vi "Extract Channel Names and Addresses from Config.vi"(0 "Config":T1={"DAQ Settings"={"Trigger Type"=enum."Manual", "Trigger Samples"=0, "Pretrigger Samples"=0, "Trigger Interval"=0.0, "Time Units"=FALSE, "Auto Save"=FALSE, "Sample Rate"=7.0, "Select Analog"=FALSE, "Trigger Value"=0.0, "Trigger Stop Method"=enum."Use Samples Value to Stop Trigger", "Rate Sec/Min"=FALSE, "Save Mode"=enum."Single File", "File Size Limit"=0.0, "Log File Type"=enum."Basic", "Trigger Data Index"=0, "Log Rate"=7.0, "Rate Sec/Min (Log)"=FALSE, "Sample Rate (S/s)"=0.0, "Log Rate (S/s)"=0.0}, "Channels"=[], "Header"={"CA Number"="", "Test Name"="", "Serial Number"="", "Technician"=""}, "Graph Settings"={"Graph Labels"=[], [], [], [], [], [], [], [], [], [], [], [], [], "Graph Toggles"=[], "Axis Toggles"=[], "Graph Range"=enum."1"}, "Test Limits"=[], "All Type Info"=[], "Save Mode"=enum."Single File", "Data Base Path"=path ""} {"DAQ Settings"."Trigger Interval" min=0.0; "DAQ Settings"."Pretrigger Samples" min=0; "DAQ Settings"."Trigger Samples" min=0}) -> (4 "Channel Names":string[](array[string]), 6 "Channel Addresses":string[](array[string]))   [LabVIEW 2023]
uses:
  Type Defs and Controls/Sensor Config.ctl
  Type Defs and Controls/DAQ Settings.ctl
  Type Defs and Controls/Trigger Stop Method.ctl
  Type Defs and Controls/Log File Type.ctl
  Type Defs and Controls/Channel Config.ctl
  Type Defs and Controls/Header.ctl
  Type Defs and Controls/Graph Settings Type Def.ctl
  Type Defs and Controls/Test Limits.ctl
  Type Defs and Controls/All Part Info.ctl
  Type Defs and Controls/Part Info.ctl
panel:
  # "EGU"
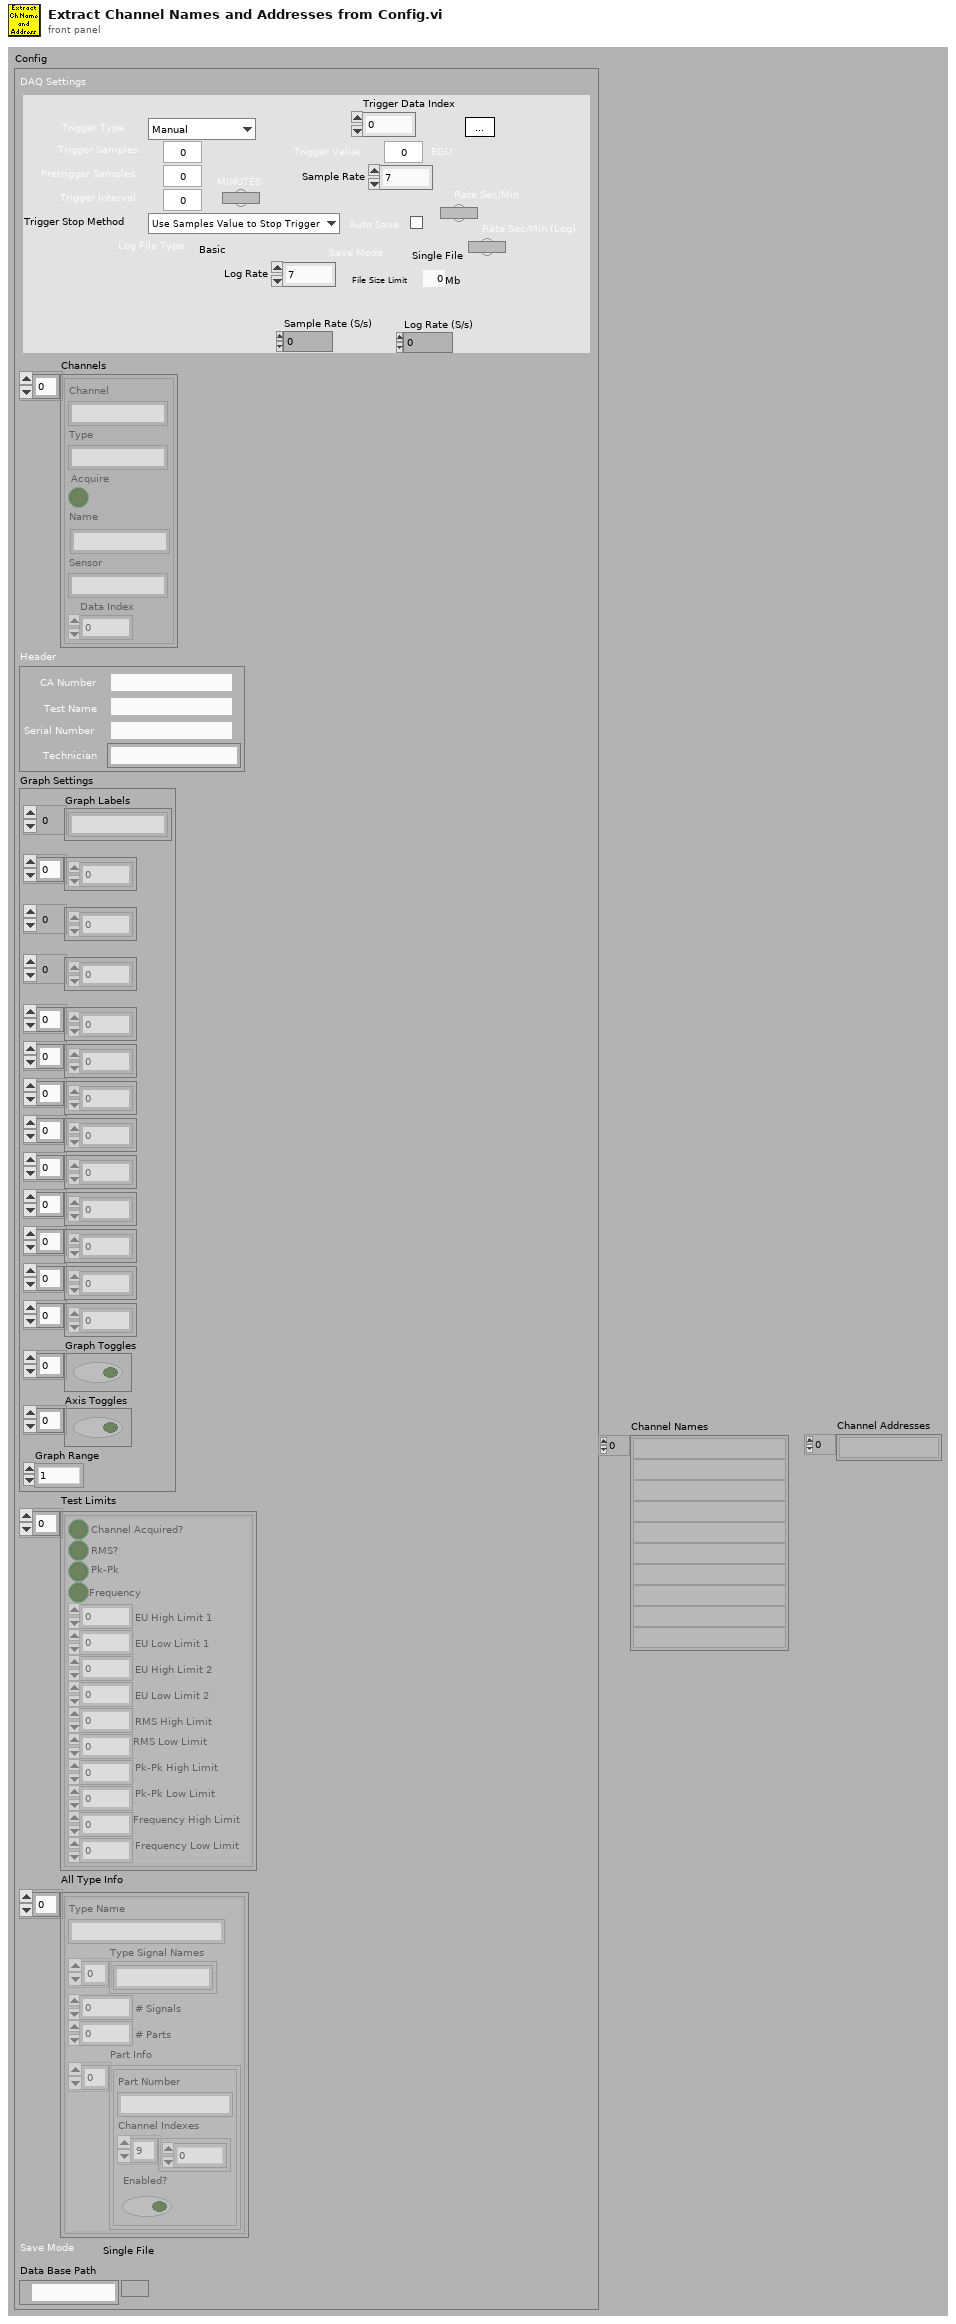
[diagram p1: front panel]
types:
  T1 = typedef "Sensor Config.ctl" = cluster{"DAQ Settings":T2, "Channels":T5[], "Header":T6, "Graph Settings":T7, "Test Limits":T8[], "All Type Info":T9, "Save Mode":enum16{"Single File", "Segmented Files", "New File at Midnight"}, "Data Base Path":path}
  T2 = typedef "DAQ Settings.ctl" = cluster{"Trigger Type":enum16{"Manual", "Timed", "Analog Rising", "Analog Falling"}, "Trigger Samples":i32, "Pretrigger Samples":i32, "Trigger Interval":dbl, "Time Units":bool, "Auto Save":bool, "Sample Rate":dbl, "Select Analog":bool, "Trigger Value":dbl, "Trigger Stop Method":T3, "Rate Sec/Min":bool, "Save Mode":enum16{"Single File", "Segmented Files", "New File at Midnight"}, "File Size Limit":dbl, "Log File Type":T4, "Trigger Data Index":u32, "Log Rate":dbl, "Rate Sec/Min (Log)":bool, "Sample Rate (S/s)":dbl, "Log Rate (S/s)":dbl}
  T3 = typedef "Trigger Stop Method.ctl" = enum16{"Use Samples Value to Stop Trigger", "Use Threshold to Stop Trigger"}
  T4 = typedef "Log File Type.ctl" = enum16{"Basic", "RTS"}
  T5 = typedef "Channel Config.ctl" = cluster{"Channel":string, "Type":string, "Acquire":bool, "Name":string, "Sensor":string, "Data Index":u32}
  T6 = typedef "Header.ctl" = cluster{"CA Number":string, "Test Name":string, "Serial Number":string, "Technician":string}
  T7 = typedef "Graph Settings Type Def.ctl" = cluster{"Graph Labels":string[], u8[], i16[], u32[], u8[], u8[], u8[], u32[], u8[], u8[], u8[], dbl[], dbl[], "Graph Toggles":bool[], "Axis Toggles":bool[], "Graph Range":enum16{"1", "2", "3", "4", "5", "10", "15", "30", "60"}}
  T8 = typedef "Test Limits.ctl" = cluster{"Channel Acquired?":bool, "RMS?":bool, "Pk-Pk":bool, "Frequency":bool, "EU High Limit 1":dbl, "EU Low Limit 1":dbl, "EU High Limit 2":dbl, "EU Low Limit 2":dbl, "RMS High Limit":dbl, "RMS Low Limit":dbl, "Pk-Pk High Limit ":dbl, "Pk-Pk Low Limit":dbl, "Frequency High Limit":dbl, "Frequency Low Limit":dbl}
  T9 = typedef "All Part Info.ctl" = cluster{"Type Name":string, "Type Signal Names":string[], "# Signals":i32, "# Parts":i32, "Part Info":T10[]}[]
  T10 = typedef "Part Info.ctl" = cluster{"Part Number":string, "Channel Indexes":u16[], "Enabled?":bool}
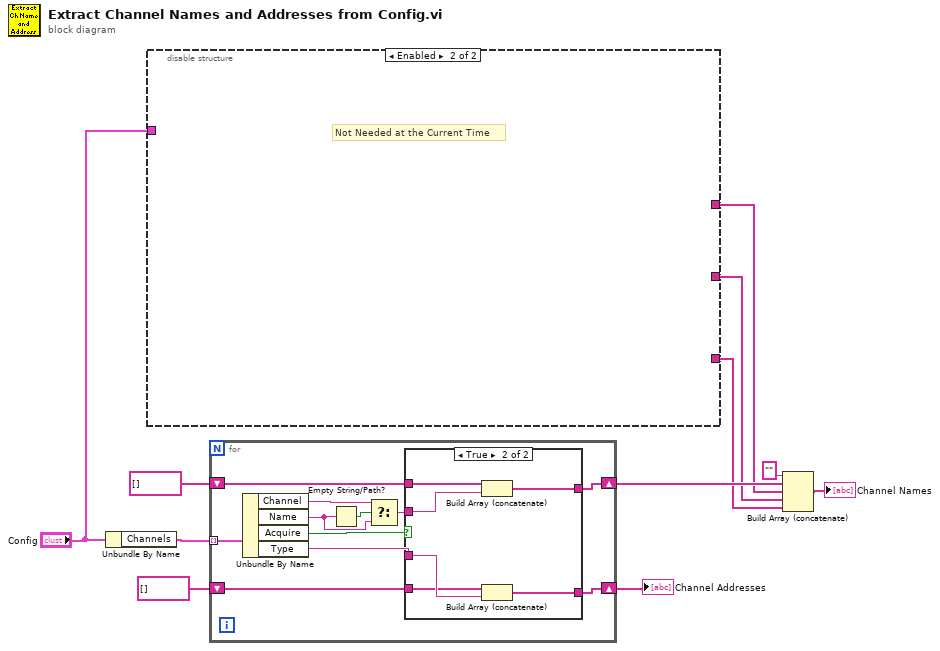
[diagram p0: block diagram]
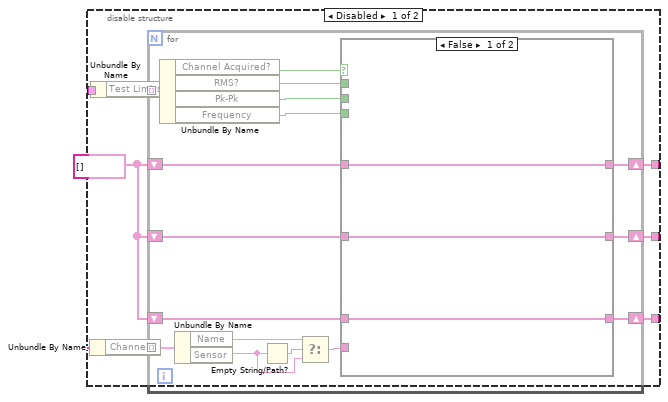
[diagram p2: hidden frame]
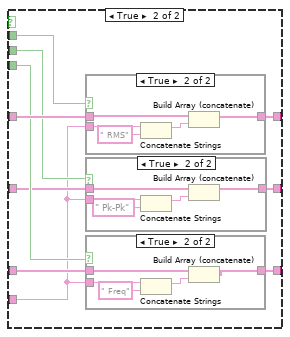
[diagram p3: hidden frame]
diagram:
  n1 = Unbundle By Name("Config") -> ("Channels"=w8:T5[])
  n2 = disable-structure shown="Enabled" {
    disable-tunnel: [w16 _] -> w5
    disable-tunnel: [w15 _] -> w4
    disable-tunnel: [w14 _] -> w3
    disable-tunnel: "Config" -> [w13 _]
    frame Disabled {
      w17 = string[] []
      n3 = Unbundle By Name(w13) -> ("Channels"=w12:T5[])
      n4 = Unbundle By Name(w13) -> ("Test Limits"=w18:T8[])
      n5 = for {
        tunnel: w18 -> [w34] mode=indexing
        shift-right: [w26] -> w16
        shift-left: w17 -> [w32]
        shift-right: [w25] -> w15
        shift-left: w17 -> [w28]
        shift-right: [w24] -> w14
        shift-left: w17 -> [w27]
        tunnel: w12 -> [w23] mode=indexing
        n6 = Unbundle By Name(w34) -> ("Channel Acquired?"=w33:bool, "RMS?"=w31:bool, "Pk-Pk"=w30:bool, "Frequency"=w29:bool)
        n7 = Unbundle By Name(w23) -> ("Name"=w20:string, "Sensor"=w21:string)
        n8 = Empty String/Path?(string/path=w21) -> (empty?=w22:bool)
        n9 = Select(t=w20, s=w22, f=w21) -> (s? t:f=w19:string)
        n10 = case shown="False" w33 {
          tunnel: w32 -> [w37 w46]
          tunnel: w31 -> [_ w47]
          tunnel: w30 -> [_ w45]
          tunnel: w29 -> [_ w44]
          tunnel: w28 -> [w36 w43]
          tunnel: w27 -> [w35 w42]
          tunnel: [w37 w41] -> w26
          tunnel: [w36 w40] -> w25
          tunnel: [w35 w39] -> w24
          tunnel: w19 -> [_ w38]
          frame False {
          }
          frame True {
            n11 = case shown="True" w47 {
              tunnel: w46 -> [w60 w65]
              tunnel: [w60 w61] -> w41
              tunnel: w38 -> [_ w64]
              frame False {
              }
              frame True {
                n12 = Concatenate Strings(w64, " RMS" ("string")) -> (w62:string)
                n13 = Build Array (concatenate)(w65, w62) -> (w61:string[])
              }
            }
            n14 = case shown="True" w45 {
              tunnel: w43 -> [w54 w57]
              tunnel: [w54 w56] -> w40
              tunnel: w38 -> [_ w55]
              frame False {
              }
              frame True {
                n15 = Concatenate Strings(w55, " Pk-Pk" ("string")) -> (w59:string)
                n16 = Build Array (concatenate)(w57, w59) -> (w56:string[])
              }
            }
            n17 = case shown="True" w44 {
              tunnel: w42 -> [w48 w51]
              tunnel: [w48 w49] -> w39
              tunnel: w38 -> [_ w50]
              frame False {
              }
              frame True {
                n18 = Concatenate Strings(w50, " Freq" ("string")) -> (w52:string)
                n19 = Build Array (concatenate)(w51, w52) -> (w49:string[])
              }
            }
          }
        }
      }
    }
    frame Enabled {
      # "Not Needed at the Current Time"
    }
  }
  n20 = for {
    tunnel: w8 -> [w76] mode=indexing
    shift-right: [w74] -> w10
    shift-left: string[] [] -> [w73]
    shift-right: [w70] -> w9
    shift-left: string[] [] -> [w71]
    n21 = Unbundle By Name(w76) -> ("Channel"=w68:string, "Name"=w67:string, "Acquire"=w75:bool, "Type"=w72:string)
    n22 = Empty String/Path?(string/path=w67) -> (empty?=w69:bool)
    n23 = Select(t=w68, s=w69, f=w67) -> (s? t:f=w66:string)
    n24 = case shown="True" w75 {
      tunnel: [w78 w84] -> w74
      tunnel: w73 -> [w78 w83]
      tunnel: w72 -> [_ w82]
      tunnel: w71 -> [w77 w81]
      tunnel: [w77 w80] -> w70
      tunnel: w66 -> [_ w79]
      frame False {
      }
      frame True {
        n25 = Build Array (concatenate)(w83, w79) -> (w84:string[])
        n26 = Build Array (concatenate)(w81, w82) -> (w80:string[])
      }
    }
  }
  "Channel Addresses" <- w9
  n27 = Build Array (concatenate)("" ("Description"), w10, w5, w4, w3) -> (→"Channel Names":string[])
